vi "BRig_dataMTrig_Laser_c_l2.vi"() -> (2 "output_Laser_c_l2":i32)   [LabVIEW 2014]
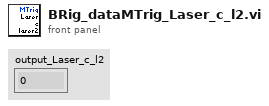
[diagram p1: front panel]
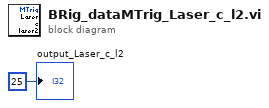
[diagram p0: block diagram]
diagram:
  "output_Laser_c_l2" <- 25 ("output_iBlock")
